vi "Measure_proc.vi"(7 "array":dbl[](array[numeric]), 8 "error in (no error)":errorcluster, 9 "Количество элементов массива":i32, 10 "Номер иттерации":i32, 11 "VISA resource name":refnum<visa-resource-name>) -> (0 "error out":errorcluster, 3 "VISA resource name out":refnum<visa-resource-name>, 4 "output array":dbl[](array[numeric]))   [LabVIEW 2018]
uses:
  <instrlib>/Tektronix DMM40x0 Series/Public/Data/Read (Single Point).vi
  <instrlib>/Tektronix DMM40x0 Series/Tektronix DMM40x0 Series.lvlib
panel:
  in  "Function (0: DC Voltage)":u16(ring) items=["DC Voltage", "AC Voltage", "2 - Wire Resistance", "4 - Wire Resistance", "DC Current", "AC Current", "Frequency", "Period", "Continuity", "Diode Checking", "Temperature", "Capacitance"]
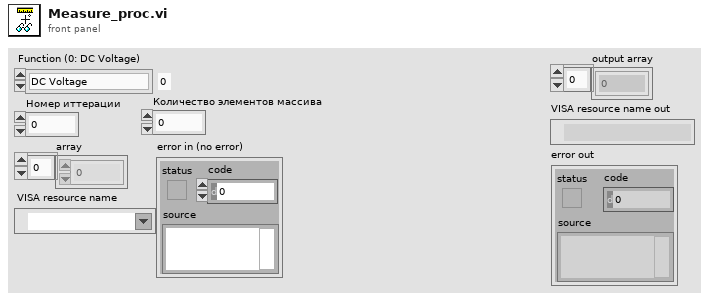
[diagram p1: front panel]
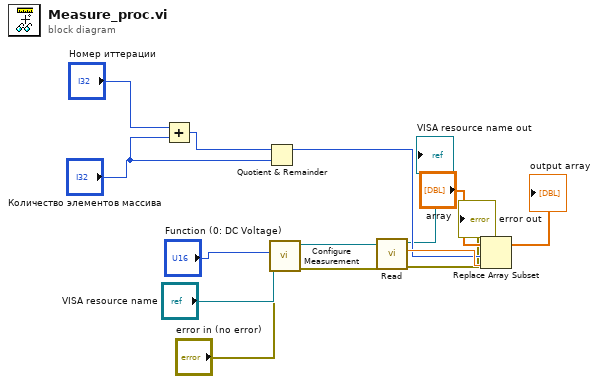
[diagram p0: block diagram]
diagram:
  n1 = Add(x="Номер иттерации", y="Количество элементов массива") -> (x+y=w10:i32)
  n2 = Quotient & Remainder(x=w10, y="Количество элементов массива") -> (x-y*floor(x/y)=w8:i32)  [unwired: 1 out]
  n3 = call <instrlib>:"Configure Measurement.vi"("error in (no error)"="error in (no error)", "Function (0: DC Voltage)"="Function (0: DC Voltage)", "VISA resource name"="VISA resource name") -> ("error out"=w3:errorcluster, "VISA resource name out"=w13:refnum<visa-resource-name>)  [unwired: 7 in]
  n4 = call-poly <instrlib>:"Read.vi"("error in (no error)"=w3, "VISA resource name"=w13) -> ("error out"=→"error out":errorcluster, "Measurement"=w12:dbl, "VISA resource name out"=→"VISA resource name out":refnum<visa-resource-name>)  [unwired: 7 in]
  n5 = Replace Array Subset(array="array", new element=w12, index=w8) -> (→"output array":dbl[])
